vi "Car Wash.vi"() -> ()   [LabVIEW 2021]
doc: "This VI allows you to simulate a car wash. The wash options controls allow you to determine which cycles will be performed. If none are selected, the High Pressure Wash cycle is the default. Once the start button is clicked, the wash begins. Use the Car Position Simulation control to simulate the position of the vehicle. If the vehicle is in the wrong position for the current cycle, the wash indicators will indicate that and you should change the car position. The Car wash display will give the current status of the wash cycle. The \"Stop Program\" button will stop the car wash immediately."
uses:
  System/bt_System.lvclass
  <vilib>/TSA/Event Log/Event_TextLog/Event_TextLog.lvclass/Event_TextLog.ctl
  <vilib>/TSA/Abstract Data Classes/Abs_Types/Boolean/Abs_Boolean.lvclass
  <vilib>/TSA/Abstract Data Classes/Abs_Types/I32 Integer/Abs_I32 Integer.lvclass
  <vilib>/TSA/Abstract Data Classes/Abs_Types/Double Float/Abs_Double Float.lvclass
  Blackboard/Blackboard.lvclass
  <vilib>/TSA/Event Log/Event_TextLog/Event_TextLog.lvclass
  Support/Car Wash Support.lvlib
panel:
  out "Log Message":string
  in  "Start":bool
  in  "Stop":bool
  out "Elapsed Time (sec)":dbl format="%#.2g"
  out "Wash Indicators":T1
  in  "Car Position Slider":i32(slide) scale=0.0..4.0
  out "Wash Entry":bool
  in  "Wash Options":T2
  # "Entry Console"
  # "Car Wash Display"
  # "The wash options controls allow you to determine which cycles will be performed.  \n\nIf none are selected, the High Pressure Wash cycle is the default.  \n\nOnce the start button is clicked, the wash begins."
  # "The Wash Entry LED indicates whether or not the wash in vacant or in use.\n\nThe Wash Indicator LEDs indicate the current status when the wash is in use.\n\nThe Elapsed Time indicator shows the progress for the current cycle, only if it is a timed cycle."
  # "Car Position Simulation"
  # "The Car Position Slider allows you to simulate the position of a vehicle in the wash.\nThe vehicle must be at the correct station for the each wash cycle to work.  The cycles that are completed at each station are indicated below the station number.\nIf the Vehicle Out of Position LED above is green, adjust your position to the appropraite station."
  # "This example is based on NI's CLD Exam Preparation Sample, linked here:\nhttps://learn.ni.com/pages/certified-labview-developer\nhttps://learn-cf.ni.com/custed/Certification/Prep%20Material/CLD/cld_sample_exams_english.zip"
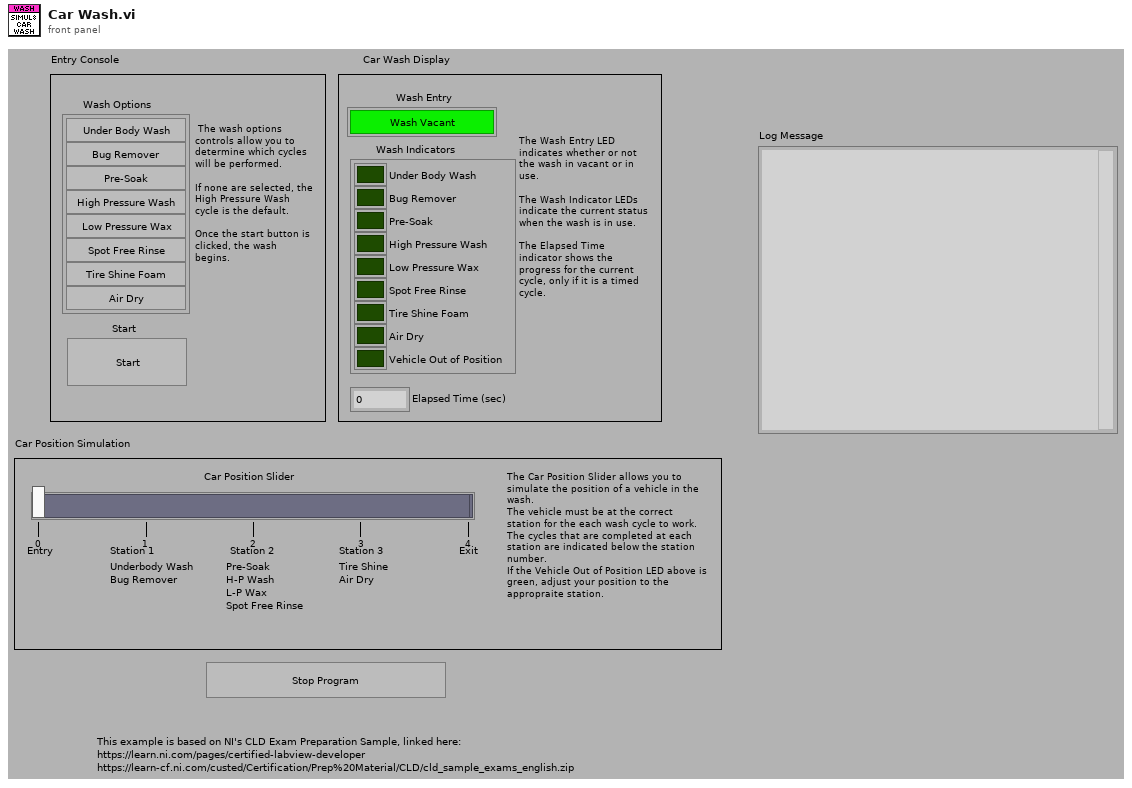
[diagram p1: front panel]
types:
  T1 = cluster{"Under Body Wash":bool, "Bug Remover":bool, "Pre-Soak":bool, "High Pressure Wash":bool, "Low Pressure Wax":bool, "Spot Free Rinse":bool, "Tire Shine Foam":bool, "Air Dry":bool, "Vehicle Out of Position":bool}
  T2 = cluster{"Under Body Wash":bool, "Bug Remover":bool, "Pre-Soak":bool, "High Pressure Wash":bool, "Low Pressure Wax":bool, "Spot Free Rinse":bool, "Tire Shine Foam":bool, "Air Dry":bool}
  T3 = typedef "Car Wash Support.lvlib/IO Refs.ctl" = cluster{"EventLog":refnum<class "Event_TextLog.lvclass">, "Wash Entry":refnum<class "Abs_Boolean.lvclass">, "Wash Indicators":T4, "Wash Options":T5, "Car Position":refnum<class "Abs_I32 Integer.lvclass">, "Elapsed Time (sec)":refnum<class "Abs_Double Float.lvclass">, "Start":refnum<class "Abs_Boolean.lvclass">}
  T4 = typedef "Car Wash Support.lvlib/Wash Indicators.ctl" = cluster{"Under Body Wash":refnum<class "Abs_Boolean.lvclass">, "Bug Remover":refnum<class "Abs_Boolean.lvclass">, "Pre-Soak":refnum<class "Abs_Boolean.lvclass">, "High Pressure Wash":refnum<class "Abs_Boolean.lvclass">, "Low Pressure Wax":refnum<class "Abs_Boolean.lvclass">, "Spot Free Rinse":refnum<class "Abs_Boolean.lvclass">, "Tire Shine Foam":refnum<class "Abs_Boolean.lvclass">, "Air Dry":refnum<class "Abs_Boolean.lvclass">, "Vehicle Out of Position":refnum<class "Abs_Boolean.lvclass">}
  T5 = typedef "Car Wash Support.lvlib/Wash Options.ctl" = cluster{"Under Body Wash":refnum<class "Abs_Boolean.lvclass">, "Bug Remover":refnum<class "Abs_Boolean.lvclass">, "Pre-Soak":refnum<class "Abs_Boolean.lvclass">, "High Pressure Wash":refnum<class "Abs_Boolean.lvclass">, "Low Pressure Wax":refnum<class "Abs_Boolean.lvclass">, "Spot Free Rinse":refnum<class "Abs_Boolean.lvclass">, "Tire Shine Foam":refnum<class "Abs_Boolean.lvclass">, "Air Dry":refnum<class "Abs_Boolean.lvclass">}
  T6 = typedef "Abs_Double Float.lvclass/Type.ctl" = dbl
  T7 = cluster{"[0]":bool, "[1]":bool, "[2]":bool, "[3]":bool, "[4]":bool, "[5]":bool, "[6]":bool, "[7]":bool, "[8]":bool}
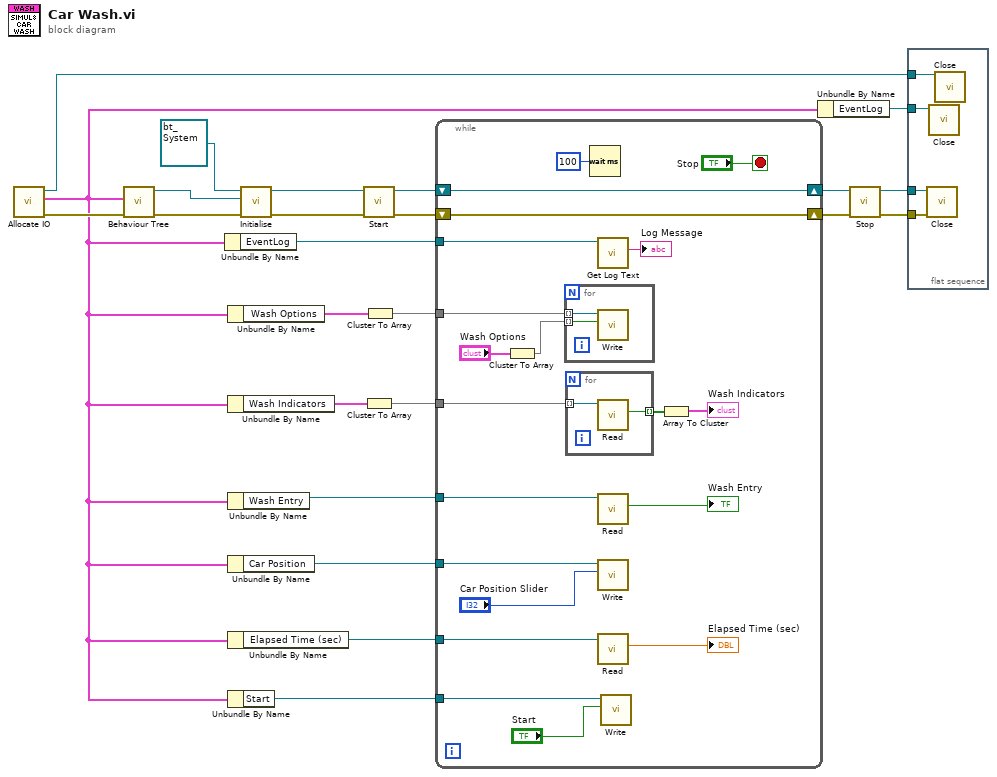
[diagram p0: block diagram]
diagram:
  n1 = call "Allocate IO.vi"() -> ("error out"=w11:errorcluster, "IO"=w2:T3, "Blackboard out"=w14:refnum<class "Blackboard.lvclass">)  [unwired: 9 in]
  n2 = call "Behaviour Tree.vi"("IO"=w2) -> ("bt_Node out"=w1:refnum<class "bt_Node.lvclass">)  [unwired: 10 in]
  n3 = Unbundle By Name(w2) -> ("EventLog"=w4:refnum<class "Event_TextLog.lvclass">)
  n4 = Unbundle By Name(w2) -> ("Wash Options"=w13:T5)
  n5 = Unbundle By Name(w2) -> ("Wash Indicators"=w12:T4)
  n6 = Unbundle By Name(w2) -> ("Wash Entry"=w9:refnum<class "Abs_Boolean.lvclass">)
  n7 = Unbundle By Name(w2) -> ("Car Position"=w7:refnum<class "Abs_I32 Integer.lvclass">)
  n8 = Unbundle By Name(w2) -> ("Elapsed Time (sec)"=w6:refnum<class "Abs_Double Float.lvclass">)
  n9 = Unbundle By Name(w2) -> ("Start"=w5:refnum<class "Abs_Boolean.lvclass">)
  n10 = call "Initialise.vi"("error in (no error)"=w11, "Behaviour Tree"=w1, "bt_System in"=refnum<class "bt_System.lvclass"> refnum) -> ("error out"=w21:errorcluster, "bt_System out"=w22:refnum<class "bt_System.lvclass">)  [unwired: 7 in]
  n11 = call "Start.vi"("error in (no error)"=w21, "bt_System in"=w22) -> ("error out"=w17:errorcluster, "bt_System out"=w20:refnum<class "bt_System.lvclass">)  [unwired: 8 in]
  n12 = Cluster To Array(cluster=w12) -> (array=w10:refnum<class "Abs_Boolean.lvclass">[])
  n13 = Cluster To Array(cluster=w13) -> (array=w8:refnum<class "Abs_Boolean.lvclass">[])
  n14 = while {
    shift-right: [w43] -> w19
    shift-left: w20 -> [w43]
    shift-right: [w42] -> w16
    shift-left: w17 -> [w42]
    tunnel: w8 -> [w39]
    tunnel: w10 -> [w41]
    tunnel: w9 -> [w35]
    tunnel: w7 -> [w31]
    tunnel: w6 -> [w28]
    tunnel: w5 -> [w27]
    tunnel: w4 -> [w25]
    stop <- "Stop" stop-if-true
    n15 = Cluster To Array(cluster="Wash Options") -> (array=w32:bool[])
    n16 = for {
      tunnel: w39 -> [w45] mode=indexing
      tunnel: w32 -> [w44] mode=indexing
      n17 = call-dynamic "Write.vi"("Boolean"=w44, "Boolean in"=w45) -> ()  [unwired: 8 in, 2 out]
    }
    n18 = for {
      tunnel: w41 -> [w47] mode=indexing
      tunnel: [w46] -> w40 mode=indexing
      n19 = call-dynamic "Read.vi"("Boolean in"=w47) -> ("Boolean"=w46:bool)  [unwired: 8 in, 2 out]
    }
    n20 = Wait (ms)(milliseconds to wait=u32 100) -> ()  [unwired: 1 out]
    n21 = call <vilib>:"Get Log Text.vi"("Event_TextLog in"=w25) -> ("Log Message"=→"Log Message":string)  [unwired: 8 in, 2 out]
    n22 = call-dynamic "Read.vi"("Boolean in"=w35) -> ("Boolean"=→"Wash Entry":bool)  [unwired: 8 in, 2 out]
    n23 = call-dynamic "Write.vi"("Value"="Car Position Slider", "Double Float.lvclass_340760 in"=w31) -> ()  [unwired: 8 in, 2 out]
    n24 = call-dynamic "Read.vi"("Double Float.lvclass_340760 in"=w28) -> ("Value"=→"Elapsed Time (sec)":T6)  [unwired: 8 in, 2 out]
    n25 = call-dynamic "Write.vi"("Boolean"="Start", "Boolean in"=w27) -> ()  [unwired: 8 in, 2 out]
    n26 = Array To Cluster(array=w40) -> (cluster=→"Wash Indicators":T7)
  }
  n27 = Unbundle By Name(w2) -> ("EventLog"=w3:refnum<class "Event_TextLog.lvclass">)
  n28 = call "Stop.vi"("error in (no error)"=w16, "bt_System in"=w19) -> ("error out"=w15:errorcluster, "bt_System out"=w18:refnum<class "bt_System.lvclass">)  [unwired: 8 in]
  n29 = flat-sequence {
    tunnel: w18 -> [w51]
    tunnel: w15 -> [w50]
    tunnel: w14 -> [w48]
    tunnel: w3 -> [w49]
    frame #0 {
      n30 = call-dynamic "Close.vi"("error in (no error)"=w50, "bt_System in"=w51) -> ()  [unwired: 8 in, 2 out]
      n31 = call-dynamic "Close.vi"("Event_TextLog in"=w49) -> ()  [unwired: 9 in, 2 out]
      n32 = call-dynamic "Close.vi"("bt_Blackboard in"=w48) -> ()  [unwired: 9 in, 2 out]
    }
  }
